vi "test Parse System Definition to Create Rx Execution Unit.vi"(8 "error in":errorcluster, 11 "TestCase in":refnum<class "Engine.lvclass">) -> (0 "error out":errorcluster, 3 "TestCase out":refnum<class "Engine.lvclass">)   [LabVIEW 2020, in "Engine.lvclass"]
uses:
  Engine.lvclass
  Shared/RT Hardware Channel Settings.ctl
  Shared/RT Label Settings.ctl
  Shared/Label.ctl
  Shared/RT Parameters.ctl
  Shared/Parameter Definition.ctl
  <vilib>/NI/NI VeriStand Encoding and Decoding/Encoding.ctl
  <vilib>/NI VeriStand/Custom Device API/Custom Device Item Ref.ctl
  Shared/Transfer Type.ctl
  <vilib>/NI VeriStand/Custom Device API/Data Reference.ctl
  Engine/Implementation/Rx Execution Unit/Rx Execution Unit.lvclass
  Engine/Implementation/Execution Unit Factory/Execution Unit Factory.lvclass
  Engine/Implementation/Rx Execution Unit/Rx Execution Unit.lvclass/Rx Execution Unit.ctl
  <vilib>/addons/_JKI Toolkits/VI Tester/TestCase.llb/TestCase.lvclass
  niveristand-custom-device-testing-tools/VeriStandTestUtilities/VeriStandTestUtilities.lvlib
  <vilib>/NI VeriStand/Custom Device API/Custom Device API.lvlib
  <vilib>/NI/NI VeriStand Encoding and Decoding/Encoding and Decoding.lvlib
  Scripting/AIM/AIM ARINC 429 Scripting.lvlib
  C:/Program Files (x86)/National Instruments/LabVIEW 2020/vi.lib/addons/_JKI Toolkits/VI Tester/TestCase.llb/TestCase.lvclass
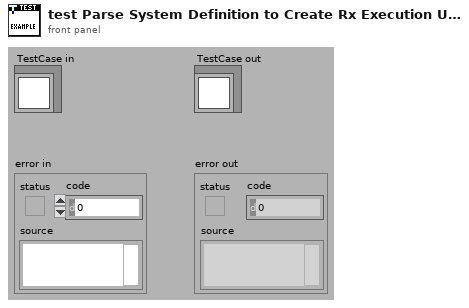
[diagram p1: front panel]
types:
  T1 = typedef "RT Hardware Channel Settings.ctl" = cluster{"channel #":u16, "channel handle":u64, "labels settings for RT":T2[]}
  T2 = typedef "RT Label Settings.ctl" = cluster{"Name":string, "xmlName":string, "label":T3, "transfer period":u32, "SDI_Enabled":bool, "SDI":u8, "parameter driver data":T4, "transfer type":T8, "has timestamp?":bool, "Label Disable/Trigger Channel Reference":T7, "Message Handle":u64, "Initialized?":bool, "Word Initial Raw Value":u32, "Label Timestamp Channel Data Reference":T9, "disabled":bool}
  T3 = typedef "Label.ctl" = u8
  T4 = typedef "RT Parameters.ctl" = cluster{"parameter definitions":T5[], "Tx parameter refs":T7[]}
  T5 = typedef "Parameter Definition.ctl" = cluster{"start index":i32, "size":i32, "encoding":T6, "signed":bool, "scale multiplier":dbl, "scale offset":dbl}
  T6 = typedef "Encoding and Decoding.lvlib/Encoding.ctl" = enum16{"BNR", "BCD", "Discrete"}
  T7 = typedef "Custom Device API.lvlib/Custom Device Item Ref.ctl" = u64
  T8 = typedef "Transfer Type.ctl" = enum16{"Scheduled", "Acyclic", "Block", "Strobe"}
  T9 = typedef "Custom Device API.lvlib/Data Reference.ctl" = i32
  T10 = typedef "AIM ARINC 429 Engine.lvlib/Interfaces.lvlib/Execution Unit Information.ctl" = cluster{"Execution Unit":refnum<class "Execution Unit.lvclass">, "Incoming Channels":T7[], "Outgoing Channels":T7[], "ReadWrite Channels":T7[]}
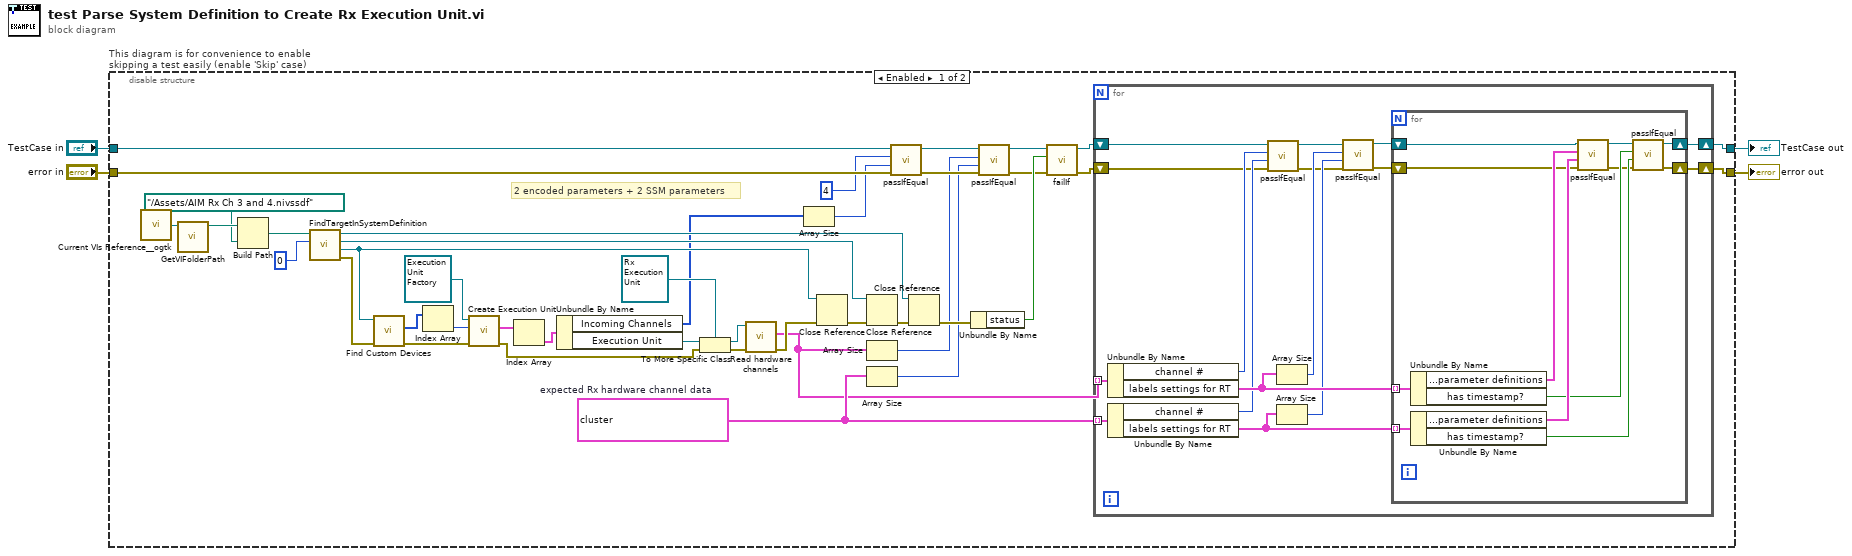
[diagram p0: block diagram]
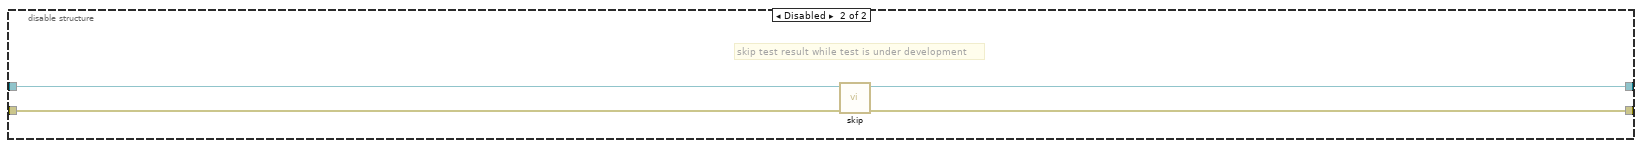
[diagram p2: hidden frame]
diagram:
  n1 = disable-structure "This diagram is for convenience to enable skipping a test easily (enable 'Skip' case)" shown="Enabled" {
    disable-tunnel: "TestCase in" -> [w46 w78]
    disable-tunnel: [w24 w76] -> w1
    disable-tunnel: [w23 w77] -> w3
    disable-tunnel: "error in" -> [w45 w75]
    frame Enabled {
      w12 = T1[] [{"channel #"=3, "channel handle"=0, "labels settings for RT"=[{"Name"="label 124", "xmlName"="", "label"=124, "transfer period"=0, "SDI_Enabled"=FALSE, "SDI"=0, "parameter driver data"={"parameter definitions"=[{"start index"=10, "size"=19, "encoding"=enum."BNR", "signed"=TRUE, "scale multiplier"=1.0, "scale offset"=0.0}, {"start index"=29, "size"=2, "encoding"=enum."BNR", "signed"=FALSE, "scale multiplier"=1.0, "scale offset"=0.0}], "Tx parameter refs"=[]}, "transfer type"=enum."Scheduled", "has timestamp?"=FALSE, "Label Disable/Trigger Channel Reference"=18446744073709551615, "Message Handle"=0, "Initialized?"=TRUE, "Word Initial Raw Value"=0, "Label Timestamp Channel Data Reference"=0, "disabled"=FALSE}]}, {"channel #"=4, "channel handle"=0, "labels settings for RT"=[{"Name"="label 125", "xmlName"="", "label"=125, "transfer period"=0, "SDI_Enabled"=FALSE, "SDI"=0, "parameter driver data"={"parameter definitions"=[{"start index"=10, "size"=19, "encoding"=enum."BNR", "signed"=TRUE, "scale multiplier"=1.0, "scale offset"=0.0}, {"start index"=29, "size"=2, "encoding"=enum."BNR", "signed"=FALSE, "scale multiplier"=1.0, "scale offset"=0.0}], "Tx parameter refs"=[]}, "transfer type"=enum."Scheduled", "has timestamp?"=FALSE, "Label Disable/Trigger Channel Reference"=18446744073709551615, "Message Handle"=0, "Initialized?"=TRUE, "Word Initial Raw Value"=0, "Label Timestamp Channel Data Reference"=0, "disabled"=FALSE}]}]  # expected Rx hardware channel data
      # "2 encoded parameters + 2 SSM parameters"
      n2 = call <userlib>:"Current VIs Reference__ogtk.vi"() -> ("Current VI's reference"=w36:refnum<vi>)  [unwired: 5 in]
      n3 = call "GetVIFolderPath.vi"("VI Reference in"=w36) -> ("VI Folder Path out"=w37:path)  [unwired: 9 in, 1 out]
      n4 = Build Path(base path=w37, name or relative path=path "../Assets/AIM Rx Ch 3 and 4.nivssdf" ("system definition path")) -> (appended path=w35:path)
      n5 = call "FindTargetInSystemDefinition.vi"("target index"=0 ("index"), "system definition path"=w35) -> ("error out"=w38:errorcluster, "Target"=w41:refnum<k24>, "Root"=w40:refnum<k24>, "System Definition"=w39:refnum<k24>)  [unwired: 6 in]
      n6 = call "Find Custom Devices.vi"("error in"=w38, "target in"=w41) -> ("error out"=w17:errorcluster, "AIM ARINC 429 custom devices"=w19:u64[])  [unwired: 7 in, 1 out]
      n7 = Index Array(array=w19) -> (element=w18:u64)  [unwired: 1 in]
      n8 = call-dynamic "Create Execution Unit.vi"("error in"=w17, "Item Ref"=w18, "Execution Unit Factory Implementation in"=refnum<class "Execution Unit Factory.lvclass"> refnum ("Communication Bus Template Interfaces:Implementation.lvlib:Execution Unit Factory.lvclass")) -> ("error out"=w7:errorcluster, "Inline Execution Units"=w16:T10[])  [unwired: 5 in, 2 out]
      n9 = Index Array(array=w16) -> (element=w15:T10)  [unwired: 1 in]
      n10 = Unbundle By Name(w15) -> ("Incoming Channels"=w5:T7[], "Execution Unit"=w14:refnum<class "Execution Unit.lvclass">)
      n11 = To More Specific Class(target class=refnum<class "Rx Execution Unit.lvclass"> refnum ("Rx Execution Unit in"), reference=w14, error in=w7) -> (specific class reference=w10:refnum<class "Rx Execution Unit.lvclass">, error out=w6:errorcluster)
      n12 = call "Read hardware channels.vi"("error in (no error)"=w6, "Rx Execution Unit in"=w10) -> ("error out"=w9:errorcluster, "hardware channels"=w8:T1[])  [unwired: 7 in, 1 out]
      n13 = Array Size(array=w5) -> (size(s)=w21:i32)
      n14 = Close Reference(reference=w41, error in (no error)=w9) -> (error out=w43:errorcluster)
      n15 = Close Reference(reference=w40, error in (no error)=w43) -> (error out=w42:errorcluster)
      n16 = Array Size(array=w8) -> (size(s)=w28:i32)
      n17 = Array Size(array=w12) -> (size(s)=w27:i32)
      n18 = call-dynamic "passIfEqual.vi"("error in (no error)"=w45, "y"=w21, "x"=4 ("size(s)"), "TestCase in"=w46) -> ("error out"=w31:errorcluster, "TestCase out"=w32:refnum<class "Engine.lvclass">)  [unwired: 6 in]
      n19 = Close Reference(reference=w39, error in (no error)=w42) -> (error out=w34:errorcluster)
      n20 = Unbundle By Name(w34) -> ("status"=w33:bool)
      n21 = call-dynamic "passIfEqual.vi"("error in (no error)"=w31, "y"=w27, "x"=w28, "TestCase in"=w32) -> ("error out"=w29:errorcluster, "TestCase out"=w30:refnum<class "Engine.lvclass">)  [unwired: 6 in]
      n22 = call-dynamic "failIf.vi"("error in (no error)"=w29, "fail"=w33, "TestCase in"=w30) -> ("error out"=w25:errorcluster, "TestCase out"=w26:refnum<class "Engine.lvclass">)  [unwired: 7 in]
      n23 = for {
        tunnel: w8 -> [w62] mode=indexing
        shift-right: [w49] -> w24
        shift-left: w26 -> [w58]
        shift-right: [w50] -> w23
        shift-left: w25 -> [w57]
        tunnel: w12 -> [w48] mode=indexing
        n24 = Unbundle By Name(w62) -> ("channel #"=w60:u16, "labels settings for RT"=w61:T2[])
        n25 = Unbundle By Name(w48) -> ("channel #"=w59:u16, "labels settings for RT"=w47:T2[])
        n26 = call-dynamic "passIfEqual.vi"("error in (no error)"=w57, "y"=w59, "x"=w60, "TestCase in"=w58) -> ("error out"=w53:errorcluster, "TestCase out"=w54:refnum<class "Engine.lvclass">)  [unwired: 6 in]
        n27 = Array Size(array=w61) -> (size(s)=w56:i32)
        n28 = Array Size(array=w47) -> (size(s)=w55:i32)
        n29 = call-dynamic "passIfEqual.vi"("error in (no error)"=w53, "y"=w55, "x"=w56, "TestCase in"=w54) -> ("error out"=w51:errorcluster, "TestCase out"=w52:refnum<class "Engine.lvclass">)  [unwired: 6 in]
        n30 = for {
          tunnel: w61 -> [w74] mode=indexing
          tunnel: w47 -> [w63] mode=indexing
          shift-right: [w65] -> w49
          shift-left: w52 -> [w67]
          shift-right: [w64] -> w50
          shift-left: w51 -> [w66]
          n31 = Unbundle By Name(w74) -> ("parameter driver data.parameter definitions"=w73:T5[], "has timestamp?"=w71:bool)
          n32 = Unbundle By Name(w63) -> ("parameter driver data.parameter definitions"=w72:T5[], "has timestamp?"=w70:bool)
          n33 = call-dynamic "passIfEqual.vi"("error in (no error)"=w66, "y"=w72, "x"=w73, "TestCase in"=w67) -> ("error out"=w68:errorcluster, "TestCase out"=w69:refnum<class "Engine.lvclass">)  [unwired: 6 in]
          n34 = call-dynamic "passIfEqual.vi"("error in (no error)"=w68, "y"=w70, "x"=w71, "TestCase in"=w69) -> ("error out"=w64:errorcluster, "TestCase out"=w65:refnum<class "Engine.lvclass">)  [unwired: 6 in]
        }
      }
    }
    frame Disabled {
      # "skip test result while test is under development"
      n35 = call <vilib>:"skip.vi"("error in (no error)"=w75, "TestCase in"=w78) -> ("error out"=w77:errorcluster, "TestCase out"=w76:refnum<class "Engine.lvclass">)  [unwired: 8 in]
    }
  }
  "error out" <- w3
  "TestCase out" <- w1
